vi "Set Frame Transfer.vi"(8 "error in (no error)":errorcluster, 11 "CCDCamera in":refnum<class "Real Camera.lvclass">) -> (0 "error out":errorcluster, 3 "CCDCamera out":refnum<class "Real Camera.lvclass">)   [LabVIEW 2018, in "Real Camera.lvclass"]
doc: "Turn the frame trasnfer mode on or off"
uses:
  Real Camera.lvclass
  C:/Users/Denis/Desktop/S4ACS/S4ACS/Simulated_CCD_Camera/Simulated Camera.lvclass
  Simulated_CCD_Camera/Simulated Camera.lvclass
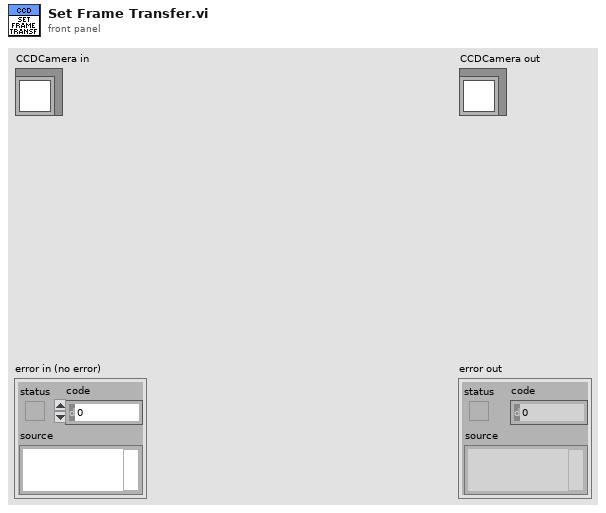
[diagram p1: front panel]
types:
  T1 = cluster{"PREAMP":u16, "READOUT_RATE":u16, "EM_GAIN":u16, "VERTICAL_SHIFT_SPEED":u16, "READ_MODE":u16, "FRAME_TRANSFER":bool, "VERTICAL_CLOCK_VOLTAGE":u16, "ACQUISITION_MODE":u16, "AD_CHANNEL":u16, "EM_MODE":u16, "SHUTTER_TTL":u16, "SHUTTER_OPENING_TIME":u16, "SHUTTER_CLOSING_TIME":u16, "SHUTTER_MODE":u16, "TRIGGER_MODE":u16, "VBIN":u16, "INITIAL_LINE":u16, "INITIAL_COLUMN":u16, "FINAL_LINE":u16, "FINAL_COLUMN":u16, "HBIN":u16}
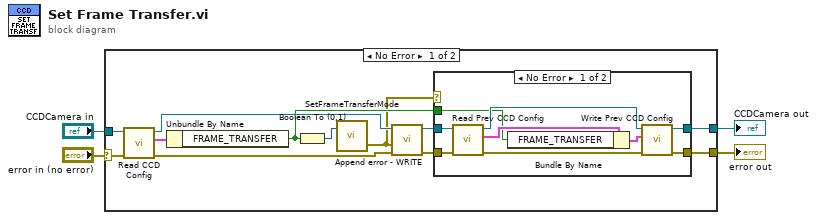
[diagram p0: block diagram]
diagram:
  n1 = case shown="No Error" "error in (no error)" {
    selector: "error in (no error)" -> [w16 w29]
    tunnel: [w8 w29] -> w4
    tunnel: [w7 w28] -> w3
    tunnel: "CCDCamera in" -> [w13 w28]
    frame No Error {
      n2 = call "Read CCD Config.vi"("error in (no error)"=w16, "CCDCamera in"=w13) -> ("error out"=w11:errorcluster, "CCD Config"=w15:T1, "CCDCamera out"=w12:refnum<class "Real Camera.lvclass">)  [unwired: 7 in]
      n3 = Unbundle By Name(w15) -> ("FRAME_TRANSFER"=w6:bool)
      n4 = Boolean To (0,1)(Boolean=w6) -> (0, 1=w14:i16)
      n5 = call <userlib>:"SetFrameTransferMode.vi"("mode"=w14) -> ("error out"=w5:errorcluster)  [unwired: 1 in, 1 out]
      n6 = call "Append error - WRITE.vi"("error in (no error)"=w11, "error"=w5, "Simulated_CCD_Camera in"=w12) -> ("error out"=w9:errorcluster, "Simulated_CCD_Camera out"=w10:refnum<class "Real Camera.lvclass">)  [unwired: 7 in]
      n7 = case shown="No Error" w5 {
        tunnel: [w24 w27] -> w7
        tunnel: [w22 w26] -> w8
        tunnel: w10 -> [w19 w27]
        tunnel: w9 -> [w17 w26]
        tunnel: w6 -> [w18 _]
        frame No Error {
          n8 = call-dynamic "Read Prev CCD Config.vi"("error in (no error)"=w17, "Simulated_CCD_Camera in"=w19) -> ("error out"=w23:errorcluster, "Prev CCD Config"=w21:T1, "Simulated_CCD_Camera out"=w25:refnum<class "Real Camera.lvclass">)  [unwired: 7 in]
          n9 = Bundle By Name(cluster=w21, "FRAME_TRANSFER"=w18) -> (w20:T1)
          n10 = call-dynamic "Write Prev CCD Config.vi"("error in (no error)"=w23, "Prev CCD Config"=w20, "Simulated_CCD_Camera in"=w25) -> ("error out"=w22:errorcluster, "Simulated_CCD_Camera out"=w24:refnum<class "Real Camera.lvclass">)  [unwired: 7 in]
        }
        frame Error {
        }
      }
    }
    frame Error {
    }
  }
  "error out" <- w4
  "CCDCamera out" <- w3
